vi "Power Create Request.vi"(8 "error in (no error)":errorcluster, 11 "Simple Reason String":string) -> (0 "error out":errorcluster, 2 "Success?":bool, 3 "Handle":i64)   [LabVIEW 2024, in "Power Requests.lvlib"]
uses:
  Power Requests.lvlib
  kernel32.dll
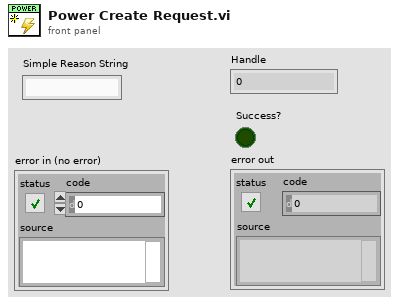
[diagram p1: front panel]
types:
  T1 = cluster{"Version":u32, "Flags":u32, "SimpleReasonString":u64}
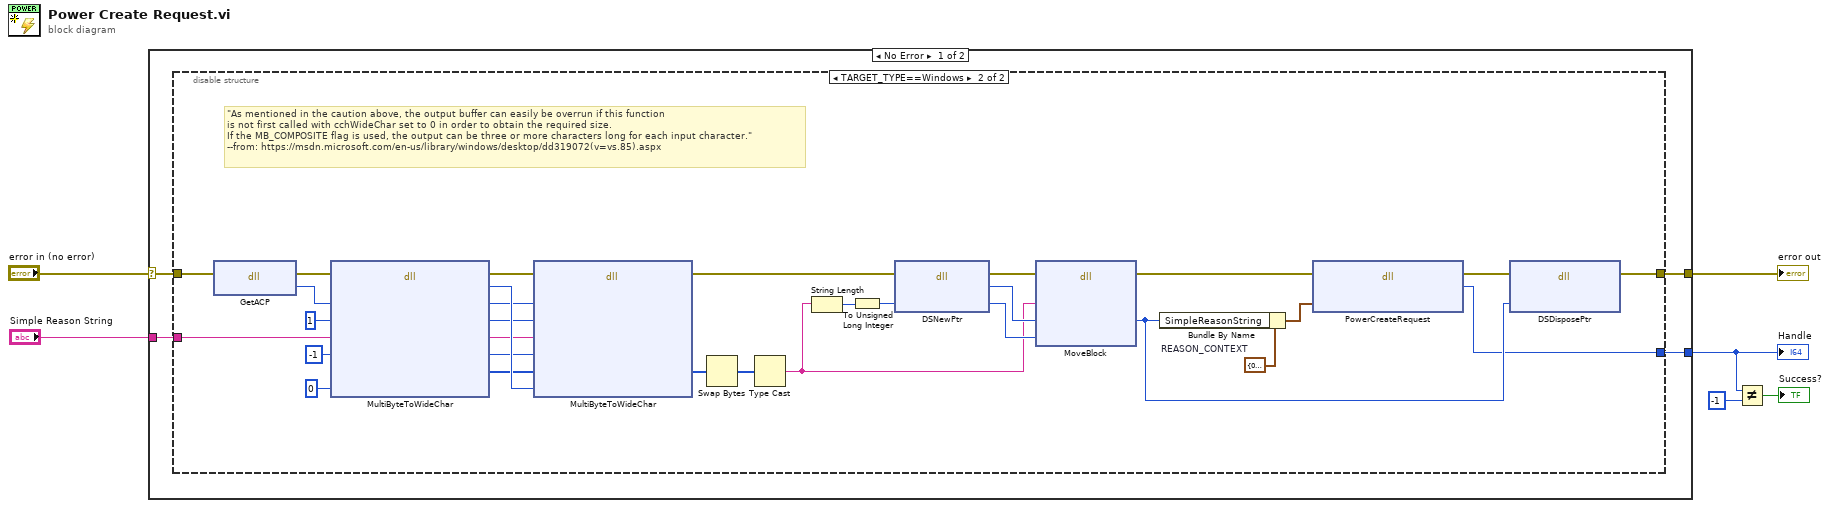
[diagram p0: block diagram]
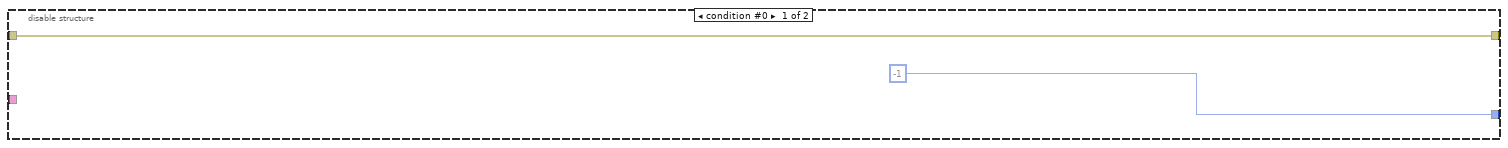
[diagram p2: hidden frame]
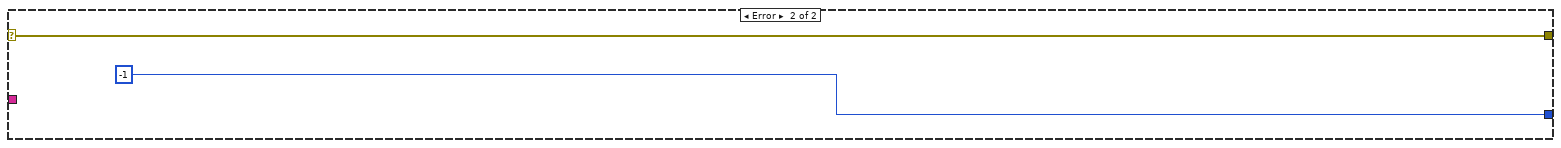
[diagram p3: hidden frame]
diagram:
  n1 = case shown="No Error" "error in (no error)" {
    selector: "error in (no error)" -> [w8 w44]
    tunnel: [w10 w44] -> w6
    tunnel: "Simple Reason String" -> [w7 _]
    tunnel: [w9 i64 -1] -> w1
    frame No Error {
      n2 = disable-structure shown="TARGET_TYPE==Windows" {
        disable-tunnel: [w12 w16] -> w10
        disable-tunnel: [i64 -1 w14] -> w9
        disable-tunnel: w8 -> [w12 w31]
        disable-tunnel: w7 -> [_ w30]
        frame condition #0 {
        }
        frame condition #1 (active) {
          w24 = T1 {"Version"=0, "Flags"=1, "SimpleReasonString"=0}  # REASON_CONTEXT
          # "\"As mentioned in the caution above, the output buffer can easily be overrun if this function\nis not first called with cchWideChar set to 0 in order to obtain the required size.\nIf the MB_COMPOSITE flag is used, the output can be three or more characters long for each input character.\"\n--from: https://msdn.microsoft.com/en-us/library/windows/desktop/dd319072(v=vs.85).aspx"
          n3 = dll-call lib="kernel32.dll" fn="GetACP" ("GetACP()")(error in=w31) -> (error out=w36:errorcluster, "UINT"=w32:u32)  [unwired: 2 in, 1 out]
          n4 = dll-call lib="kernel32.dll" fn="MultiByteToWideChar"(error in=w36, "_In_ CodePage"=w32, "_In_ dwFlags"=u32 1 ("MB_PRECOMPOSED"), "_In_ lpMultByteStr"=w30, "_In_ cbMultByte"=-1 ("nChars"), "_In_ cchWideChar"=0 ("nWStr")) -> (error out=w37:errorcluster, "INT"=w42:i32, "_In_ CodePage"=w38:u32, "_In_ dwFlags"=w39:u32, "_In_ lpMultByteStr"=w40:string, "_In_ cbMultByte"=w41:i32, "_Out_opt_ lpWideCharStr"=w13:u16[])  [unwired: 4 in, 1 out]
          n5 = dll-call lib="kernel32.dll" fn="MultiByteToWideChar"(error in=w37, "_In_ CodePage"=w38, "_In_ dwFlags"=w39, "_In_ lpMultByteStr"=w40, "_In_ cbMultByte"=w41, "_Out_opt_ lpWideCharStr"=w13, "_In_ cchWideChar"=w42) -> (error out=w26:errorcluster, "_Out_opt_ lpWideCharStr"=w22:u16[])  [unwired: 8 in, 1 out]
          n6 = Swap Bytes(anything=w22) -> (byte swapped=w19:u16[])
          n7 = Type Cast(x=w19) -> (*(type *) &x=w21:string)  [unwired: 1 in]
          n8 = String Length(string=w21) -> (length=w18:i32)
          n9 = To Unsigned Long Integer(number=w18) -> (unsigned 32bit integer=w20:u32)
          n10 = dll-call lib="LabVIEW" fn="DSNewPtr"(error in=w26, "size"=w20) -> (error out=w29:errorcluster, "return type"=w27:u64, "size"=w28:u32)  [unwired: 2 in, 1 out]
          n11 = dll-call lib="LabVIEW" fn="MoveBlock"(error in=w29, "pSrc"=w21, "pDst"=w27, "size"=w28) -> (error out=w25:errorcluster, "pDst"=w15:u64)  [unwired: 5 in, 1 out]
          n12 = Bundle By Name(cluster=w24, "SimpleReasonString"=w15) -> (w23:T1)
          n13 = dll-call lib="kernel32.dll" fn="PowerCreateRequest"(error in=w25, "_In_ PREASON_CONTEXT"=w23) -> (error out=w17:errorcluster, "HANDLE"=w14:i64)  [unwired: 3 in, 1 out]
          n14 = dll-call lib="LabVIEW" fn="DSDisposePtr"(error in=w17, "Pointer"=w15) -> (error out=w16:errorcluster)  [unwired: 4 in, 1 out]
        }
      }
    }
    frame Error {
    }
  }
  "error out" <- w6
  "Handle" <- w1
  n15 = Not Equal?(x=w1, y=i64 -1) -> (x != y?=→"Success?":bool)
